vi "read.vi"(7 "msTimeout":i32, 8 "error in (no error)":errorcluster caption="错误输入（无错误）", 9 "count":i32, 10 "data":u8[](array[numeric]), 11 "handle":u64) -> (0 "error out":errorcluster caption="错误输出", 1 "count out":i32, 2 "data out":u8[](array[numeric]), 3 "handle out":u64, 5 "function return":i32)   [LabVIEW 2018, in "InstrumentsPlayground.lvlib"]
doc: "CLIFFAPI int read(FT_HANDLE handle, uchar *data, int *count, int msTimeout=0);"
uses:
  InstrumentsPlayground.lvlib
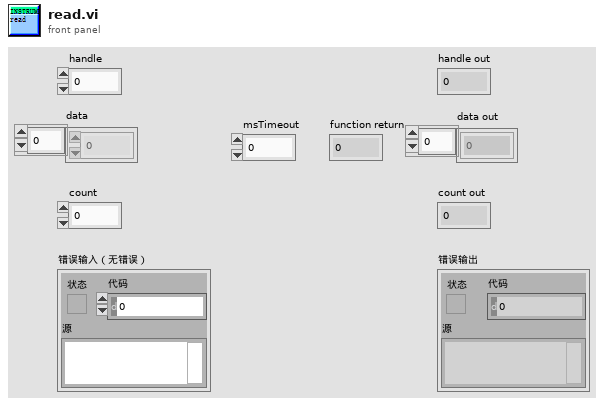
[diagram p1: front panel]
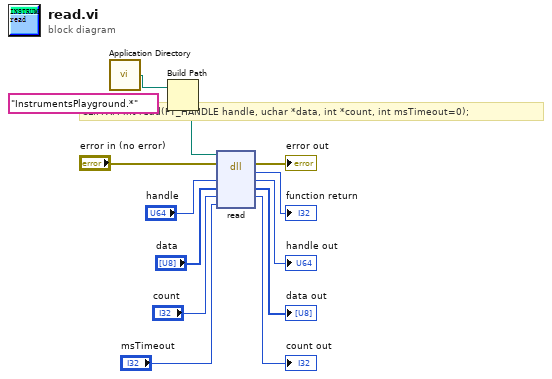
[diagram p0: block diagram]
diagram:
  # "CLIFFAPI int read(FT_HANDLE handle, uchar *data, int *count, int msTimeout=0);"
  n1 = call <vilib>:"Application Directory.vi"() -> ("Application Directory"=w2:path)
  n2 = Build Path(base path=w2, name or relative path="InstrumentsPlayground.*" ("名称或相对路径")) -> (appended path=w1:path)
  n3 = dll-call lib="E:/work/YZCourse_Xtext/Cliff/API/IPLabView lib/InstrumentsPlayground.*" fn="read"(path in=w1, error in="error in (no error)", "handle"="handle", "data"="data", "count"="count", "msTimeout"="msTimeout") -> (error out=→"error out":errorcluster, "返回类型"=→"function return":i32, "handle"=→"handle out":u32, "data"=→"data out":u8[], "count"=→"count out":i32)  [unwired: 2 in, 1 out]
